vi "HB.vi"(8 "error in (no error)":errorcluster) -> (0 "error out":errorcluster)   [LabVIEW 2018, in "MQTT Messages.lvlib"]
uses:
  MQTT Messages.lvlib
  MQTT_Singleton/MQTT_Singleton.lvlib
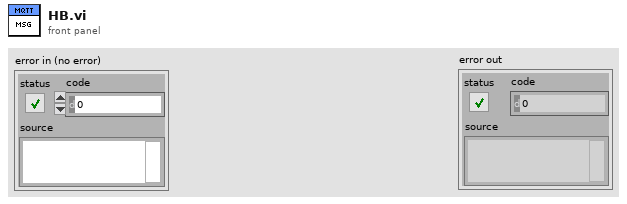
[diagram p1: front panel]
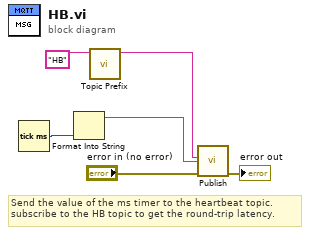
[diagram p0: block diagram]
diagram:
  # "Send the value of the ms timer to the heartbeat topic.\nsubscribe to the HB topic to get the round-trip latency."
  n1 = Tick Count (ms)() -> (millisecond timer value=w4:u32)
  n2 = Format Into String(w4) -> (resulting string=w3:string)  [unwired: 3 in, 1 out]
  n3 = call "Topic Prefix.vi"("Topic"="HB" ("string")) -> ("Topic"=w1:string)  [unwired: 9 in, 1 out]
  n4 = call "Publish.vi"("error in (no error)"="error in (no error)", "Message"=w3, "Topic"=w1) -> ("error out"=→"error out":errorcluster)  [unwired: 8 in]
